vi "Dashboard Main.vi"() -> ()   [LabVIEW 2018]
uses:
  <vilib>/Utility/miscctls.llb/LVRowAndColumnTypeDef.ctl
  <vilib>/event_ctls.llb/eventvkey.ctl
  <vilib>/Rock Robotics/Network Tables/NT Read Boolean Array.vi
  <vilib>/Rock Robotics/Network Tables/NT Read Numeric Array.vi
  <vilib>/Rock Robotics/Network Tables/NT Write Numeric Array.vi
  <vilib>/Rock Robotics/Network Tables/NT Write Boolean.vi
  <vilib>/Rock Robotics/Network Tables/NT Write String Array.vi
  <vilib>/Rock Robotics/WPI/Dashboard/WPI_DashboardLogging Global.vi
panel:
  in  "Camera Name":string(combo)="No Camera Selection"
  in  "Camera Settings Right":T1={"Frame Rate"=30, "Compression"=30, "Size"=1, "DB Camera Config"=FALSE} {"Frame Rate" scale=1.0..30.0; "Compression" scale=100.0..-1.0; "Size" items=["640x480", "320x240", "160x120"]}
  in  "Camera Name Right":string(combo)="No Camera Selection"
  out "Camera Perf":string
  in  "Camera Settings":T1={"Frame Rate"=30, "Compression"=30, "Size"=1, "DB Camera Config"=FALSE} {"Frame Rate" scale=1.0..30.0; "Compression" scale=100.0..-1.0; "Size" items=["640x480", "320x240", "160x120"]}
  in  "TCP":refnum<k5>
  in  "Rec Mode":enum32{"Stop", "Record", "Playback"}(radio)
  out "Robot IP":string
  out "Image Message":string="Timeout in Camera Communications"
  in  "Dashboard Tab":T2(tab)
  out "SideOfFieldIndicator":bool
  in  "Side of Field:":string(combo)
  in  "Camera Lights Off:":bool
  out "Error Message:":string
  in  "Run Automated:":bool
  out "NT Connection":bool
  out "Mode":T3(ring)=enum."Auto Disabled"
  out "Right Camera Perf":cluster{"Bandwidth (Mbps)":dbl, "FPS":dbl}
  out "Front Left Setpoint:":dbl(knob)
  out "Front Right Setpoint:":dbl(knob)
  out "Back Left Setpoint:":dbl(knob)
  out "Back Right Setpoint:":dbl(knob)
  out "Reversed Modules":bool[](array[boolean])
  in  "Write Swerve Offsets:":bool
  in  "Task:":string(combo)
  out "PositionIndicator":bool
  out "TaskIndicator":bool
  in  "Start Position:":string(combo)
  out "Camera Image Right":T4(plugin-control)
  in  "CheckList":i32(listbox)
  in  "Test Slider":dbl(slide) scale=0.0..100.0 scale format="%#_3g"
  in  "On/Off":bool caption="Solenoid"
  in  "Test Name":u16(ring) items=["Select the test to run..."]
  in  "Test Tree":string(tree)
  in  "Motor":cluster{"Value":dbl, "Enable":bool} {"Value" scale=-1.0..1.0 scale format="%#_3g"}
  out "Progress":T5 {"Test Progress" scale=0.0..100.0}
  in  "Rev/Fwd":cluster{"Forward":bool, "Reverse":bool}
  in  "Test Ring":u16(ring) items=["Monochrome", "Color"]
  out "Cmd Status":string
  in  "Execute Command":bool
  in  "Command Params":string[][](table)
  in  "Command Selection":i32(listbox)
  out "Tree":string(tree)
  out "Camera Image":T4(plugin-control)
  out "Background":bool
  # "HW"
  # "HW"
  # "Swerve Modules:"
  # "Sandstorm Options:"
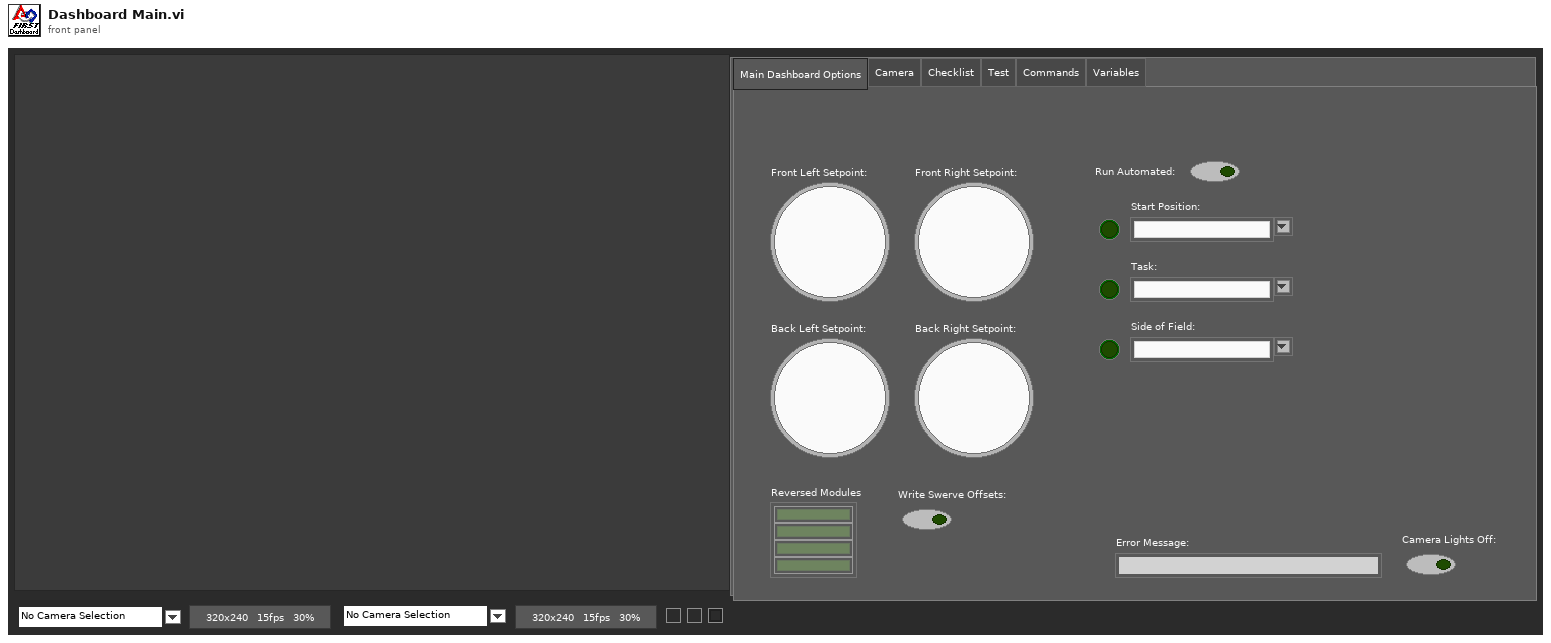
[diagram p1: front panel]
types:
  T1 = cluster{"Frame Rate":i32, "Compression":i32, "Size":u16, "DB Camera Config":bool}
  T2 = enum32{"Main Dashboard Options", "Camera", "Checklist", "Test", "Commands", "Variables"}
  T3 = enum8{"Tele-Op Disabled", "Tele-Op Enabled", "Auto Disabled", "Auto Enabled", "Test Disabled", "Test Enabled", "Disconnected", "No Code", "E-Stop"}
  T4 = typedef "IMAQ Image.ctl" = refnum<image>
  T5 = cluster{"Test Progress":u8, "Test Progress Text":string}
  T6 = cluster{"Save Path":path, "Interval (s)":dbl, "Keep":i32}
  T7 = enum32{"Drive", "Camera", "Basic", "Custom", "Test", "Commands", "Checklist", "Variables"}
  T8 = typedef "Image Type" = u32
  T9 = cluster{"IDs":cluster{"RPC field ID":u16, "Unique ID":u16}, "String":string}
  T10 = enum16{"open", "replace", "create", "open or create", "replace or create", "replace or create with confirmation"}
  T11 = cluster{"Error Strings":string, "Disable Counts":cluster{u16, u16}, "Rail Faults":cluster{u16, u16, u16}, "Robot IP":string, "DB Mode":u8, "Event Info":cluster{"Name":string, "Type":u8, "Number":u16, "Replay":u8}}
  T12 = cluster{"Storage":cluster{"Disk Free":u64, "RAM Block":u32, "RAM free":u32}, "CPU Utilization":cluster{"CPU % ISR":sgl, "CPU % Time Crit":sgl, "CPU % Timed Str":sgl, "CPU % High":sgl, "CPU % Above":sgl, "CPU % Normal":sgl, "CPU % Low":sgl}, "CAN":cluster{"% Bus Utilization":sgl, "Bus Off Cnt":u32, "TX_FIFO Full Cnt":u32, "Receive Error Cnt":u8, "Transmit Error Cnt":u8}, "HID":cluster{"HID Outputs":u32, "Rumble Low":u16, "Rumble High":u16}[]}
  T13 = cluster{"Status bits":cluster{"Test Mode":bool, "Autonomous":bool, "Enabled":bool, "Code Start":bool, "Brownout":bool, "Reserved 2":bool, "Reserved 3":bool, "E-Stop":bool}, "Code Trace":cluster{"Disabled":bool, "TeleOp":bool, "Auto":bool, "Test":bool}, "Controller Type":enum16{"unknown", "cRIO", "roboRio"}, "Code?":enum16{"unknown", "noCode", "code"}, "Battery V":dbl}
  T14 = cluster{"Control Bits":cluster{"TestMode":bool, "Autonomous":bool, "Enabled":bool, "FMS Present":bool, bool, bool, bool, "E-Stop":bool}, "Team Station ":u8, "Countdown":sgl, "Joystick Values":cluster{"Axes":dbl[], "Buttons":bool[], "POVs":i16[]}[]}
  T15 = cluster{"Camera Image":refnum<vi>, "Dashboard Tab":refnum<vi>, "Background":refnum<vi>, "Rec Mode":refnum<vi>, "Test Slider":refnum<vi>, "On/Off ":refnum<vi>, "Test Ring":refnum<vi>, "Rev/Fwd":refnum<vi>, "Test Name":refnum<vi>, "Motor":refnum<vi>, "Progress":refnum<vi>, "CheckList":refnum<vi>, "Tree":refnum<vi>, "Test Tree":refnum<vi>, "Command Params":refnum<vi>, "Command Selection":refnum<vi>, "Execute Command":refnum<vi>, "Cmd Status":refnum<vi>, "Camera Settings":refnum<vi>, "Camera Name":refnum<vi>, "Camera Perf":refnum<vi>, "Camera Settings Right":refnum<vi>, "Camera Name Right":refnum<vi>, "Camera Image Right":refnum<vi>}
  T16 = cluster{"Global Rectangle":i32[], "Contours":cluster{"Contour Type":u32, "ROI Type":u32, "Points":i32[]}[]}
  T17 = cluster{"Camera Name":string, string, "Saved DB Images Info":cluster{"Save Path":path, "Interval (s)":dbl, "Keep":i32}}
  T18 = cluster{"Camera Name Right":string, string, "Saved DB Images Info":cluster{"Save Path":path, "Interval (s)":dbl, "Keep":i32}}
  T19 = cluster{"Operation":enum16{"Update", "Clear"}, "Color Box":u32}[]
  T20 = typedef "eventvkey.ctl" = enum16{"ASCII", "Enter", "Return", "Shift", "Ctrl", "Alt", "Cmd", "Opt", "Caps", "NumLock", "Clear", "Break", "Up", "Down", "Left", "Right", "Insert", "Delete", "Home", "End", "PageUp", "PageDown", "Escape", "Help", "Pause", "ScrollLock", "F1", "F2", "F3", "F4", "F5", "F6", "F7", "F8", "F9", "F10", "F11", "F12", "F13", "F14", "F15", "F16", "F17", "F18", "F19", "F20", "F21", "F22", "F23", "F24", "Play", "VolumeUp", "VolumeDown", "Mute", "Two Byte Char"}
  T21 = cluster{"Image Size":bool, "Image Type":bool, "Pixel Value":bool, "ROI Information":bool, "Zoom Factor":bool}
  T22 = cluster{"Operation":enum16{"Update", "Clear"}, "Color Box":u32}
  T23 = typedef "LVRowAndColumnTypeDef.ctl" = cluster{"Row":i32, "Column":i32}
  T24 = cluster{"Shift":bool, "Ctrl":bool, "Alt":bool, "Cmd":bool, "Opt":bool}
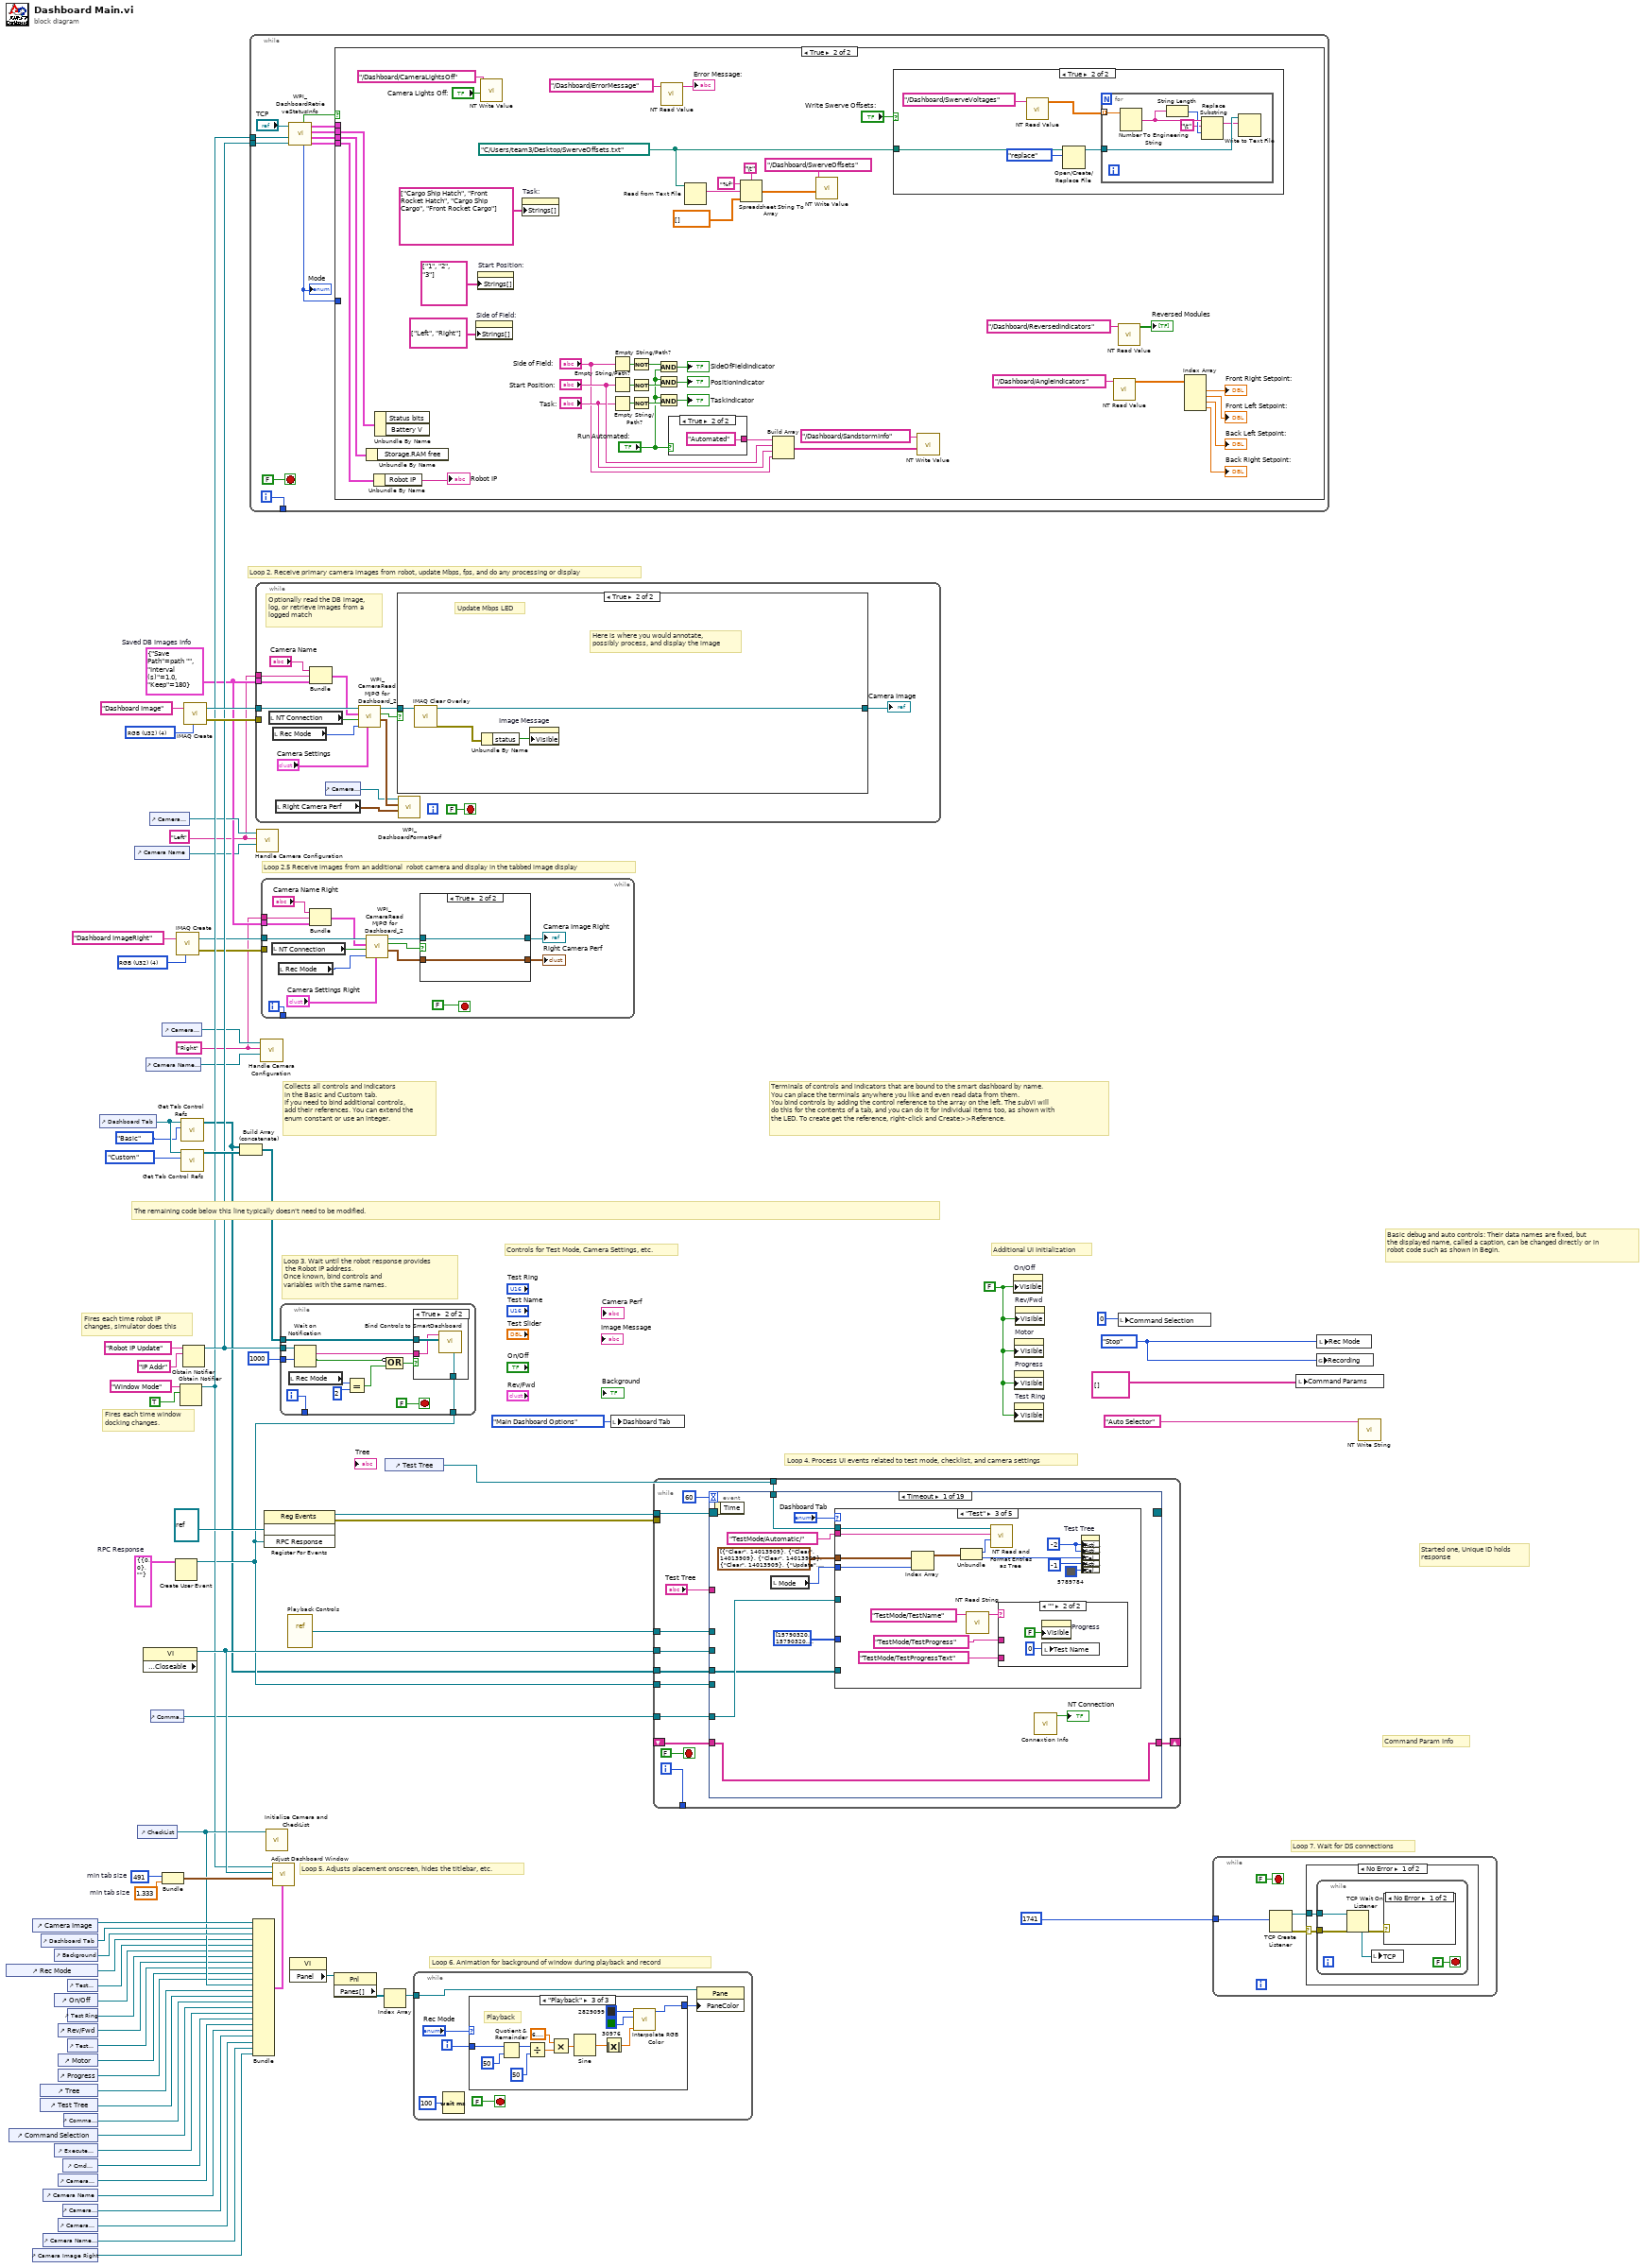
[diagram p0: block diagram]
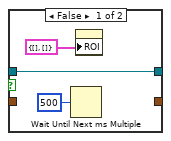
[diagram p2: hidden frame]
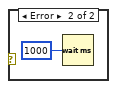
[diagram p3: hidden frame]
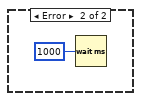
[diagram p4: hidden frame]
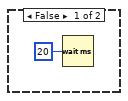
[diagram p5: hidden frame]
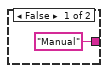
[diagram p6: hidden frame]
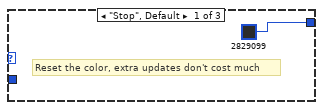
[diagram p8: hidden frame]
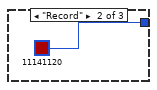
[diagram p9: hidden frame]
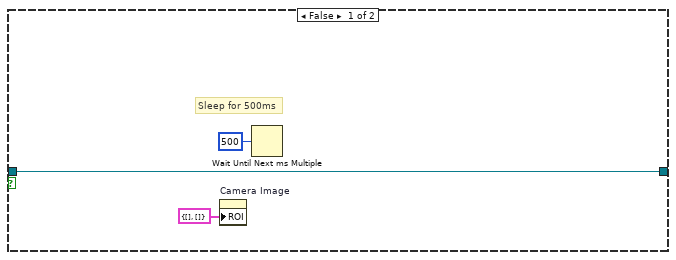
[diagram p11: hidden frame]
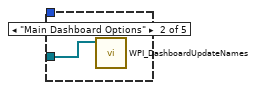
[diagram p13: hidden frame]
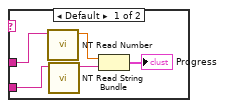
[diagram p14: hidden frame]
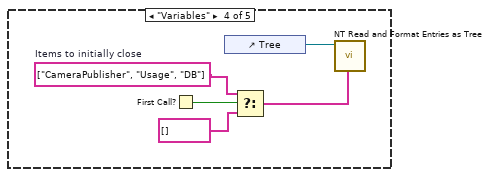
[diagram p15: hidden frame]
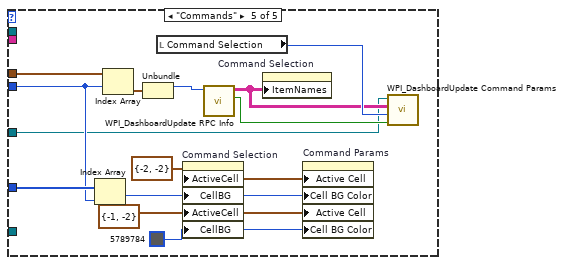
[diagram p16: hidden frame]
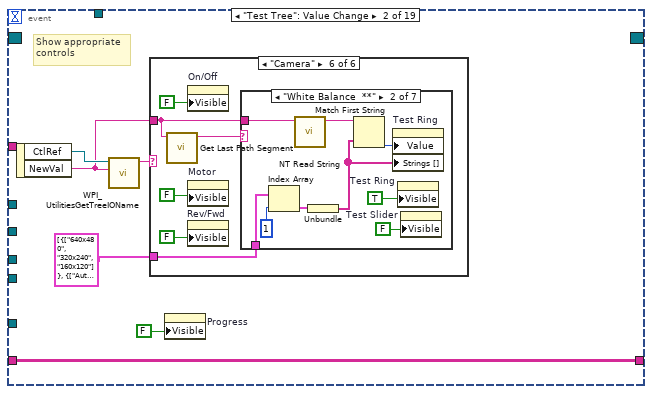
[diagram p17: hidden frame]
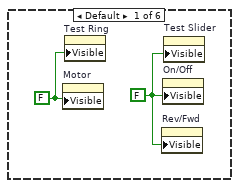
[diagram p18: hidden frame]
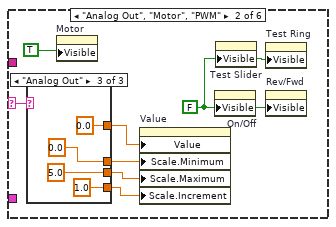
[diagram p19: hidden frame]
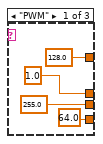
[diagram p20: hidden frame]
diagram:
  w6 = T6 {"Save Path"=path "", "Interval (s)"=1.0, "Keep"=180}  # Saved DB Images Info
  w5 = "Right"
  w4 = "Left"
  w16 = T8 4 items=["Grayscale (U8)", "Grayscale (I16)", "Grayscale (SGL)", "Complex (CSG)", "RGB (U32)", "HSL (U32)", "RGB (U64)"] ("Image Type")
  w29 = T9 {"IDs"={"RPC field ID"=0, "Unique ID"=0}, "String"=""}  # RPC Response
  w51 = 491  # min tab size
  w50 = 1.333  # min tab size
  w58 = enum32{"Stop", "Record", "Playback"}."Stop" ("Rec Mode")
  w35 = FALSE ("Visible")
  w75 = T8 4 items=["Grayscale (U8)", "Grayscale (I16)", "Grayscale (SGL)", "Complex (CSG)", "RGB (U32)", "HSL (U32)", "RGB (U64)"] ("Image Type")
  # "Loop 2.5 Receive images from an additional  robot camera and display in the tabbed image display"
  # "Command Param Info"
  # "Started one, Unique ID holds\nresponse"
  # "Loop 7. Wait for DS connections"
  # "Basic debug and auto controls: Their data names are fixed, but\nthe displayed name, called a caption, can be changed directly or in\nrobot code such as shown in Begin."
  # "Controls for Test Mode, Camera Settings, etc."
  # "Additional UI Initialization"
  # "Loop 6. Animation for background of window during playback and record"
  # "Fires each time robot IP\nchanges, simulator does this"
  # "Fires each time window\ndocking changes."
  # "Collects all controls and indicators\nin the Basic and Custom tab.\nIf you need to bind additional controls,\nadd their references. You can extend the\nenum constant or use an integer."
  # "The remaining code below this line typically doesn't need to be modified."
  # "Loop 4. Process UI events related to test mode, checklist, and camera settings"
  # "Terminals of controls and indicators that are bound to the smart dashboard by name.\nYou can place the terminals anywhere you like and even read data from them.\nYou bind controls by adding the control reference to the array on the left. The subVI will\ndo this for the contents of a tab, and you can do it for individual items too, as shown with\nthe LED. To create get the reference, right-click and Create>>Reference."
  # "Loop 3. Wait until the robot response provides\n the Robot IP address.\nOnce known, bind controls and\nvariables with the same names."
  # "Loop 5. Adjusts placement onscreen, hides the titlebar, etc."
  # "Loop 2. Receive primary camera images from robot, update Mbps, fps, and do any processing or display"
  n1 = control-ref of="Rec Mode"() -> (w41:refnum<vi>)
  n2 = control-ref of="Command Selection"() -> (w28:refnum<vi>)
  n3 = control-ref of="Camera Image"() -> (w53:refnum<vi>)
  n4 = control-ref of="Camera Image Right"() -> (w9:refnum<vi>)
  n5 = control-ref of="Tree"() -> (w45:refnum<vi>)
  n6 = control-ref of="Test Tree"() -> (w44:refnum<vi>)
  n7 = control-ref of="Dashboard Tab"() -> (w52:refnum<vi>)
  n8 = control-ref of="Camera Name"() -> (w2:refnum<vi>)
  n9 = control-ref of="Camera Name Right"() -> (w10:refnum<vi>)
  n10 = control-ref of="Background"() -> (w48:refnum<vi>)
  n11 = control-ref of="On/Off"() -> (w39:refnum<vi>)
  n12 = control-ref of="Execute Command"() -> (w30:refnum<vi>)
  n13 = control-ref of="Rev/Fwd"() -> (w37:refnum<vi>)
  n14 = control-ref of="Motor"() -> (w42:refnum<vi>)
  n15 = control-ref of="Progress"() -> (w36:refnum<vi>)
  n16 = control-ref of="Camera Settings"() -> (w21:refnum<vi>)
  n17 = control-ref of="Camera Settings Right"() -> (w11:refnum<vi>)
  n18 = control-ref of="Cmd Status"() -> (w24:refnum<vi>)
  n19 = control-ref of="Camera Perf"() -> (w20:refnum<vi>)
  n20 = control-ref of="Command Params"() -> (w31:refnum<vi>)
  n21 = control-ref of="Test Slider"() -> (w40:refnum<vi>)
  n22 = control-ref of="Test Ring"() -> (w38:refnum<vi>)
  n23 = control-ref of="Test Name"() -> (w43:refnum<vi>)
  n24 = control-ref of="Dashboard Tab"() -> (w56:refnum<vi>)
  n25 = control-ref of="Camera Name"() -> (w3:refnum<vi>)
  n26 = control-ref of="CheckList"() -> (w46:refnum<vi>)
  n27 = property class="VI" props=["Front Panel.Closeable"]() -> (reference out=w57:refnum<vi>)  [unwired: 2 in, 2 out]
  n28 = control-ref of="Camera Name Right"() -> (w12:refnum<vi>)
  n29 = control-ref of="Camera Settings"() -> (w22:refnum<vi>)
  n30 = control-ref of="Command Params"() -> (w23:refnum<vi>)
  n31 = control-ref of="Camera Settings Right"() -> (w13:refnum<vi>)
  n32 = Bundle("min tab size"=w51, "min tab size"=w50) -> (w49:cluster{"min tab size":i32, "min tab size":dbl})  [unwired: 1 in]
  n33 = Create User Event(user event datatype=w29) -> (user event=w25:refnum<user-event>)  [unwired: 1 in, 1 out]
  n34 = call "IMAQ Create"("Image Name"="Dashboard ImageRight", "Image Type"=w16) -> ("New Image"=w15:T4, "error out"=w14:errorcluster)  [unwired: 2 in, 1 out]
  n35 = Obtain Notifier(name (unnamed)="Window Mode", notification data type=TRUE) -> (notifier out=w33:refnum<notifier>)  [unwired: 2 in, 2 out]
  n36 = call <vilib>:"Get Tab Control Refs.vi"("Page Index"=T7."Basic" ("Dashboard Tab"), "TabControl in"=w56) -> ("ControlsOnPage"=w19:refnum<vi>[])  [unwired: 9 in]
  n37 = call <vilib>:"Get Tab Control Refs.vi"("Page Index"=T7."Custom" ("Dashboard Tab"), "TabControl in"=w56) -> ("ControlsOnPage"=w55:refnum<vi>[])  [unwired: 9 in]
  n38 = Obtain Notifier(name (unnamed)="Robot IP Update", notification data type="IP Addr" ("name (unnamed)")) -> (notifier out=w34:refnum<notifier>)  [unwired: 2 in, 2 out]
  n39 = call "IMAQ Create"("Image Name"="Dashboard Image", "Image Type"=w75) -> ("New Image"=w73:T4, "error out"=w72:errorcluster)  [unwired: 2 in, 1 out]
  n40 = Build Array (concatenate)(w19, w55) -> (w54:refnum<vi>[])
  n41 = while {
    tunnel: [w85] -> _
    tunnel: w34 -> [w79]
    tunnel: w33 -> [w76]
    i -> [w85]
    stop <- FALSE stop-if-true
    n42 = call <vilib>:"WPI_DashboardRetrieveStatusInfo.vi"("Binding Refnum"=w79, "Window Mode Notifier"=w76, "TCP Cnx"="TCP") -> ("Power and Errors"=w80:T11, "Robot Metrics"=w83:T12, "Status Info"=w84:T13, "Control Info"=w81:T14, "Robot Mode"=w78:T3, "Process?"=w82:bool)  [unwired: 3 in]
    "Mode" <- w78
    n43 = case shown="True" w82 {
      tunnel: w84 -> [_ w130]
      tunnel: w83 -> [_ w129]
      tunnel: w81 -> [_ _]
      tunnel: w80 -> [_ w128]
      tunnel: w78 -> [_ _]
      frame False {
        n44 = Wait (ms)(milliseconds to wait=u32 20) -> ()  [unwired: 1 out]
      }
      frame True {
        w110 = path "C:/Users/team3/Desktop/SwerveOffsets.txt" ("file (use dialog)")
        n45 = Unbundle By Name(w129) -> ()  [unwired: 1 out]
        n46 = Unbundle By Name(w128) -> ("Robot IP"=→"Robot IP":string)
        n47 = Unbundle By Name(w130) -> ()  [unwired: 2 out]
        n48 = property on="Side of Field:" class="CmbBox"("Strings[]"=string[] ["Left", "Right"]) -> ()  [unwired: 2 in, 2 out]
        n49 = property on="Start Position:" class="CmbBox"("Strings[]"=string[] ["1", "2", "3"]) -> ()  [unwired: 2 in, 2 out]
        n50 = call-poly <vilib>:"NT Write Value.vi"("Boolean"="Camera Lights Off:", "Name"="/Dashboard/CameraLightsOff") -> ()  [unwired: 9 in, 1 out]
        n51 = property on="Task:" class="CmbBox"("Strings[]"=string[] ["Cargo Ship Hatch", "Front Rocket Hatch", "Cargo Ship Cargo", "Front Rocket Cargo"]) -> ()  [unwired: 2 in, 2 out]
        n52 = Empty String/Path?(string/path="Side of Field:") -> (empty?=w91:bool)
        n53 = Empty String/Path?(string/path="Start Position:") -> (empty?=w106:bool)
        n54 = Empty String/Path?(string/path="Task:") -> (empty?=w103:bool)
        n55 = Not(x=w91) -> (.not. x?=w89:bool)
        n56 = Not(x=w106) -> (.not. x?=w105:bool)
        n57 = Not(x=w103) -> (.not. x?=w104:bool)
        n58 = And(x=w89, y="Run Automated:") -> (x .and. y?=→"SideOfFieldIndicator":bool)
        n59 = And(x="Run Automated:", y=w105) -> (x .and. y?=→"PositionIndicator":bool)
        n60 = And(x="Run Automated:", y=w104) -> (x .and. y?=→"TaskIndicator":bool)
        n61 = call-poly <vilib>:"NT Read Value.vi"("Name"="/Dashboard/ErrorMessage") -> ("String"=→"Error Message:":string)  [unwired: 9 in, 1 out]
        n62 = case shown="True" "Run Automated:" {
          tunnel: ["Manual" "Automated"] -> w100
          frame False {
          }
          frame True {
          }
        }
        n63 = Read from Text File(file (use dialog)=w110) -> (text=w124:string)  [unwired: 3 in, 3 out]
        n64 = Spreadsheet String To Array(delimiter (Tab)="\t", format string="%f", spreadsheet string=w124, array type (2D Dbl)=dbl[] []) -> (array=w123:dbl[])
        n65 = Build Array(w100, "Start Position:", "Task:", "Side of Field:") -> (w107:string[])
        n66 = call-poly <vilib>:"NT Write Value.vi"("Numeric Array"=w123, "Name"="/Dashboard/SwerveOffsets") -> ()  [unwired: 9 in, 1 out]
        n67 = case shown="True" "Write Swerve Offsets:" {
          tunnel: w110 -> [_ w134]
          frame False {
          }
          frame True {
            n68 = call-poly <vilib>:"NT Read Value.vi"("Name"="/Dashboard/SwerveVoltages") -> ("Numeric Array"=w133:dbl[])  [unwired: 9 in, 1 out]
            n69 = Open/Create/Replace File(file path (use dialog)=w134, operation (0:open)=T10."replace") -> (refnum out=w136:refnum<file>)  [unwired: 4 in, 2 out]
            n70 = for {
              tunnel: w136 -> [w142]
              tunnel: w133 -> [w143] mode=indexing
              n71 = Number To Engineering String(4:w143) -> (0:w141:string)  [unwired: 3 in]
              n72 = String Length(string=w141) -> (length=w140:i32)
              n73 = Replace Substring(3:w140, 4:"\t", 5:w141) -> (1:w138:string)  [unwired: 1 in, 1 out]
              n74 = Write to Text File(file (use dialog)=w142, text=w138) -> ()  [unwired: 2 in, 3 out]
            }
          }
        }
        n75 = call-poly <vilib>:"NT Write Value.vi"("String Array"=w107, "Name"="/Dashboard/SandstormInfo") -> ()  [unwired: 9 in, 1 out]
        n76 = call-poly <vilib>:"NT Read Value.vi"("Name"="/Dashboard/AngleIndicators") -> ("Numeric Array"=w115:dbl[])  [unwired: 9 in, 1 out]
        n77 = call-poly <vilib>:"NT Read Value.vi"("Name"="/Dashboard/ReversedIndicators") -> ("Boolean Array"=→"Reversed Modules":bool[])  [unwired: 9 in, 1 out]
        n78 = Index Array(array=w115) -> (element #1=→"Front Right Setpoint:":dbl, element #2=→"Front Left Setpoint:":dbl, element #3=→"Back Left Setpoint:":dbl, element #4=→"Back Right Setpoint:":dbl)  [unwired: 4 in]
      }
    }
  }
  n79 = Bundle("Camera Image"=w53, "Dashboard Tab"=w52, "Background"=w48, "Rec Mode"=w41, "Test Slider"=w40, "On/Off"=w39, "Test Ring"=w38, "Rev/Fwd"=w37, "Test Name"=w43, "Motor"=w42, "Progress"=w36, "CheckList"=w46, "Tree"=w45, "Test Tree"=w44, "Command Params"=w31, "Command Selection"=w28, "Execute Command"=w30, "Cmd Status"=w24, "Camera Settings"=w21, "Camera Name"=w2, "Camera Perf"=w20, "Camera Settings Right"=w11, "Camera Name Right"=w10, "Camera Image Right"=w9) -> (w47:T15)  [unwired: 1 in]
  n80 = while {
    tunnel: w73 -> [w157]
    tunnel: w72 -> [_]
    tunnel: w6 -> [w150]
    tunnel: w4 -> [w148]
    stop <- FALSE stop-if-true
    # "Optionally read the DB image,\nlog, or retrieve images from a\nlogged match"
    n81 = local read "NT Connection"() -> (w151:bool)
    n82 = local read "Rec Mode"() -> (w154:enum32{"Stop", "Record", "Playback"})
    n83 = local read "Right Camera Perf"() -> (w146:cluster{"Bandwidth (Mbps)":dbl, "FPS":dbl})
    n84 = Bundle("Camera Name"="Camera Name", w148, "Saved DB Images Info"=w150) -> (w149:T17)  [unwired: 1 in]
    n85 = control-ref of="Camera Perf"() -> (w145:refnum<vi>)
    n86 = call <vilib>:"WPI_CameraRead MJPG for Dashboard_2.vi"("Camera Settings"="Camera Settings", "Rec Mode"=w154, "NT Connection"=w151, "Capture Info"=w149, "Image in"=w157) -> ("perf info"=w147:cluster{"Bandwidth (Mbps)":dbl, "fps":dbl}, "Active"=w155:bool, "Image\\ out"=w156:T4)  [unwired: 4 in]
    n87 = case shown="True" w155 {
      tunnel: w156 -> [w160 w163]
      tunnel: [w160 w162] -> w152
      frame False {
        # "Sleep for 500ms"
        n88 = property on="Camera Image" class="ImageControl"("ROI"=T16 {"Global Rectangle"=[], "Contours"=[]}) -> ()  [unwired: 2 in, 2 out]
        n89 = Wait Until Next ms Multiple(millisecond multiple=u32 500) -> ()  [unwired: 1 out]
      }
      frame True {
        # "Here is where you would annotate,\npossibly process, and display the image"
        # "Update Mbps LED"
        n90 = call "IMAQ Clear Overlay"("Image"=w163) -> ("error out"=w164:errorcluster, "Image Out"=w162:T4)  [unwired: 2 in, 7 out]
        n91 = Unbundle By Name(w164) -> ("status"=w165:bool)
        n92 = property on="Image Message" class="Str"("Visible"=w165) -> ()  [unwired: 2 in, 2 out]
      }
    }
    "Camera Image" <- w152
    n93 = call <vilib>:"WPI_DashboardFormatPerf.vi"("Right Camera Perf"=w146, "Performance"=w147, "String in"=w145) -> ()  [unwired: 9 in]
  }
  n94 = call "Handle Camera Configuration.vi"("CameraNameRef"=w3, "Display Name"=w4, "ClusterRef"=w22) -> ()  [unwired: 9 in]
  n95 = call "Handle Camera Configuration.vi"("CameraNameRef"=w12, "Display Name"=w5, "ClusterRef"=w13) -> ()  [unwired: 9 in]
  n96 = while {
    tunnel: w15 -> [w180]
    tunnel: w14 -> [_]
    tunnel: [w175] -> _
    tunnel: w6 -> [w171]
    tunnel: w5 -> [w168]
    i -> [w175]
    stop <- FALSE stop-if-true
    n97 = local read "NT Connection"() -> (w172:bool)
    n98 = local read "Rec Mode"() -> (w179:enum32{"Stop", "Record", "Playback"})
    n99 = Bundle("Camera Name Right"="Camera Name Right", w168, "Saved DB Images Info"=w171) -> (w170:T18)  [unwired: 1 in]
    n100 = call <vilib>:"WPI_CameraRead MJPG for Dashboard_2.vi"("Camera Settings"="Camera Settings Right", "Rec Mode"=w179, "NT Connection"=w172, "Capture Info"=w170, "Image in"=w180) -> ("perf info"=w166:cluster{"Bandwidth (Mbps)":dbl, "fps":dbl}, "Active"=w174:bool, "Image\\ out"=w177:T4)  [unwired: 4 in]
    n101 = case shown="True" w174 {
      tunnel: w177 -> [w182 w185]
      tunnel: [w182 w185] -> w173
      tunnel: [_ w184] -> w167
      tunnel: w166 -> [_ w184]
      frame False {
        n102 = Wait Until Next ms Multiple(millisecond multiple=u32 500) -> ()  [unwired: 1 out]
        n103 = property on="Camera Image Right" class="ImageControl"("ROI"=T16 {"Global Rectangle"=[], "Contours"=[]}) -> ()  [unwired: 2 in, 2 out]
      }
      frame True {
      }
    }
    "Camera Image Right" <- w173
    "Right Camera Perf" <- w167
  }
  n104 = register-events(refnum<vi> refnum, w25) -> (reference out=w62:refnum<event-registration>, error out=w61:errorcluster)  [unwired: 2 in]
  n105 = call "Initialize Camera and CheckList.vi"("ListBox in"=w46) -> ()  [unwired: 11 in]
  n106 = call "Adjust Dashboard Window.vi"("Sizing Refnums"=w47, "Size Constraints"=w49, "VI"=w57, "WIn Mode"=w33) -> ()  [unwired: 8 in]
  n107 = while {
    tunnel: w54 -> [w197]
    tunnel: w34 -> [w195]
    tunnel: [w193] -> _
    tunnel: u32 1000 ("milliseconds to wait") -> [w192]
    tunnel: w25 -> [w186]
    i -> [w193]
    stop <- FALSE stop-if-true
    n108 = local read "Rec Mode"() -> (w188:enum32{"Stop", "Record", "Playback"})
    n109 = Wait on Notification(notifier=w195, timeout in ms (-1)=w192) -> (notification=w194:string, timed out?=w190:bool)  [unwired: 2 in, 2 out]
    n110 = Equal?(x=w188, y=u16 2 ("Rec Mode")) -> (x = y?=w189:bool)
    n111 = Compound Arithmetic op=OR(invert w190, w189) -> (w191:bool)
    n112 = case shown="True" w191 {
      tunnel: w197 -> [_ w200]
      tunnel: w194 -> [_ w199]
      tunnel: w186 -> [_ w198]
      frame False {
      }
      frame True {
        n113 = call <vilib>:"Bind Controls to SmartDashboard.vi"("RPC ref"=w198, "Bound Control Refs"=w200, "Server IP Address"=w199) -> ()  [unwired: 9 in]
      }
    }
  }
  n114 = vi-ref "Playback Controls.vi"() -> (w63:refnum<vi>)
  n115 = property class="VI"() -> ("Panel"=w65:refnum<vi>)  [unwired: 2 in, 2 out]
  n116 = property class="Pnl"(reference=w65) -> ("Panes[]"=w66:refnum<vi>[])  [unwired: 1 in, 2 out]
  n117 = Index Array(array=w66) -> (element=w64:refnum<vi>)  [unwired: 1 in]
  n118 = control-ref of="Test Tree"() -> (w67:refnum<vi>)
  n119 = while {
    tunnel: w64 -> [w202]
    i -> [w205]
    stop <- FALSE stop-if-true
    n120 = Wait (ms)(milliseconds to wait=u32 100) -> ()  [unwired: 1 out]
    n121 = case shown="\"Playback\"" "Rec Mode" {
      tunnel: w205 -> [_ _ w220]
      tunnel: [u32 2829099 ("Base Color") u32 11141120 ("Target Color") w209] -> w201
      frame "Stop", Default {
        # "Reset the color, extra updates don't cost much"
      }
      frame "Record" {
      }
      frame "Playback" {
        # "Playback"
        n122 = Quotient & Remainder(x=w220, y=u32 50 ("milliseconds to wait")) -> (x-y*floor(x/y)=w216:u32)  [unwired: 1 out]
        n123 = Divide(x=w216, y=u32 50 ("milliseconds to wait")) -> (x/y=w213:dbl)
        n124 = Multiply(x=6.283185307179586, y=w213) -> (x*y=w218:dbl)
        n125 = Sine(x=w218) -> (sin(x)=w217:dbl)
        n126 = Absolute Value(x=w217) -> (abs(x)=w210:dbl)
        n127 = call "Interpolate RGB Color.vi"("Proportion"=w210, "Target Color"=u32 30976, "Base Color"=u32 2829099) -> ("Result Color"=w209:u32)  [unwired: 8 in]
      }
    }
    n128 = property class="Pane"(reference=w202, "PaneColor"=w201) -> ()  [unwired: 1 in, 2 out]
  }
  n129 = local write "Dashboard Tab"(T2."Main Dashboard Options" ("Dashboard Tab")) -> ()
  n130 = while {
    tunnel: [w230] -> _
    tunnel: w67 -> [w229]
    tunnel: w63 -> [w228]
    tunnel: w62 -> [w227]
    tunnel: w61 -> [_]
    tunnel: w57 -> [w226]
    tunnel: w25 -> [w225]
    tunnel: w23 -> [w224]
    shift-right: [w223] -> _
    shift-left: _ -> [w222]
    tunnel: w19 -> [w221]
    i -> [w230]
    stop <- FALSE stop-if-true
    n131 = event shown="[0] Timeout" {
      selector: w227 -> [_ _ _ _ _ _ _ _ _ _ _ _ _ _ _ _ _ _ _]
      dyn-events: [_ _ _ _ _ _ _ _ _ _ _ _ _ _ w484 _ _ _ _] -> _
      timeout: u32 60 ("milliseconds to wait") -> [_ _ _ _ _ _ _ _ _ _ _ _ _ _ _ _ _ _ _]
      tunnel: w229 -> [w242 _ _ _ _ _ _ _ _ _ _ _ _ _ _ _ _ _ _]
      tunnel: "Test Tree" -> [_ _ _ _ _ _ _ _ _ w451 w459 w461 w465 w473 _ _ _ _ _]
      tunnel: w228 -> [_ _ _ _ _ _ _ _ _ _ _ _ _ _ w486 _ w504 _ _]
      tunnel: w226 -> [_ _ _ _ _ _ _ _ _ _ _ _ _ _ w482 _ _ _ _]
      tunnel: w225 -> [_ _ _ _ _ _ _ _ _ _ _ _ _ _ w480 _ _ _ _]
      tunnel: w224 -> [w237 _ _ _ w402 _ _ _ _ _ _ _ _ _ _ _ _ _ _]
      tunnel: [w236 w285 w387 w392 w400 w409 w419 w426 w438 w450 w457 w460 w464 w472 w479 w499 w501 w505 w518] -> w223
      tunnel: w222 -> [w236 w285 w387 w392 w400 _ _ w426 w438 w450 w457 w460 w464 w472 w479 w499 w501 w505 w518]
      tunnel: w221 -> [w234 _ _ _ _ _ _ _ _ _ _ _ _ _ _ _ _ _ _]
      event Timeout {
        n132 = event-data() -> ()  [unwired: 1 in, 1 out]
        n133 = local read "Mode"() -> (w239:T3)
        n134 = case shown="\"Test\"" "Dashboard Tab" {
          tunnel: w242 -> [_ _ w258 _ _]
          tunnel: "TestMode/Automatic/" ("Name Pattern") -> [_ _ w257 _ _]
          tunnel: T19 [{"Operation"=enum."Clear", "Color Box"=14013909}, {"Operation"=enum."Clear", "Color Box"=14013909}, {"Operation"=enum."Clear", "Color Box"=14013909}, {"Operation"=enum."Clear", "Color Box"=14013909}, {"Operation"=enum."Update", "Color Box"=14013909}, {"Operation"=enum."Update", "Color Box"=16777215}, {"Operation"=enum."Clear", "Color Box"=14013909}, {"Operation"=enum."Clear", "Color Box"=14013909}, {"Operation"=enum."Clear", "Color Box"=14013909}] -> [_ _ w250 _ w278]
          tunnel: w239 -> [_ _ w249 _ w277]
          tunnel: u32[] [15790320, 15790320, 15790320, 15790320, 16777215, 16777215, 15790320, 15790320, 15790320] -> [_ _ _ _ w283]
          tunnel: w237 -> [_ _ _ _ w271]
          tunnel: w234 -> [_ w244 _ _ _]
          frame "Camera", Default {
          }
          frame "Main Dashboard Options" {
            n135 = call <vilib>:"WPI_DashboardUpdateNames.vi"("Controls on Tab"=w244) -> ()  [unwired: 11 in]
          }
          frame "Test" {
            w256 = -2 ("Active Item:Row Number")
            n136 = Index Array(array=w250, index=w249) -> (element=w251:T22)
            n137 = Unbundle(w251) -> ("Operation"=w252:enum16{"Update", "Clear"}, "Color Box"=w253:u32)
            n138 = call <vilib>:"NT Read String.vi"("Name"="TestMode/TestName") -> ("String"=w247:string)  [unwired: 9 in, 1 out]
            n139 = call <vilib>:"NT Read and Format Entries as Tree.vi"("Operation"=w252, "Name Pattern"=w257, "Tree Refnum"=w258) -> ()  [unwired: 7 in, 2 out]
            n140 = case shown="\"\"" w247 {
              tunnel: "TestMode/TestProgress" ("Name") -> [w260 _]
              tunnel: "TestMode/TestProgressText" ("Name") -> [w259 _]
              frame Default {
                n141 = call <vilib>:"NT Read Number.vi"("Name"=w260) -> ("Numeric"=w261:dbl)  [unwired: 9 in, 1 out]
                n142 = call <vilib>:"NT Read String.vi"("Name"=w259) -> ("String"=w262:string)  [unwired: 9 in, 1 out]
                n143 = Bundle("Numeric"=w261, "String"=w262) -> (→"Progress":cluster{"Numeric":dbl, "String":string})  [unwired: 1 in]
              }
              frame "" {
                n144 = property on="Progress" class="Clust (strict)"("Visible"=FALSE) -> ()  [unwired: 2 in, 2 out]
                n145 = local write "Test Name"(u16 0) -> ()
              }
            }
            n146 = property on="Test Tree" class="Tree (strict)"("Active Item Row Number"=w256, "ActiveColNum"=w256, "CellBG"=w253, "Active Item Row Number"=-1 ("Active Item:Row Number"), "CellBG"=u32 5789784 ("Color Box")) -> ()  [unwired: 2 in, 2 out]
          }
          frame "Variables" {
            w268 = string[] ["CameraPublisher", "Usage", "DB"]  # Items to initially close
            n147 = First Call?() -> (First Call?: T/F=w269:bool)
            n148 = control-ref of="Tree"() -> (w270:refnum<vi>)
            n149 = Select(t=w268, s=w269, f=string[] []) -> (s? t:f=w266:string[])
            n150 = call <vilib>:"NT Read and Format Entries as Tree.vi"("Tags to  Close"=w266, "Tree Refnum"=w270) -> ()  [unwired: 8 in, 2 out]
          }
          frame "Commands" {
            w279 = u32 5789784 ("Color Box")
            w280 = T23 {"Row"=-1, "Column"=-2} ("Active Cell:Active Cell")
            w282 = T23 {"Row"=-2, "Column"=-2} ("Active Cell:Active Cell")
            n151 = Index Array(array=w283, index=w277) -> (element=w281:u32)
            n152 = Index Array(array=w278, index=w277) -> (element=w276:T22)
            n153 = Unbundle(w276) -> ("Operation"=w275:enum16{"Update", "Clear"})  [unwired: 1 out]
            n154 = local read "Command Selection"() -> (w274:i32)
            n155 = property on="Command Selection" class="MCListbox (strict)"("ActiveCell"=w282, "CellBG"=w281, "ActiveCell"=w280, "CellBG"=w279) -> ()  [unwired: 2 in, 2 out]
            n156 = call <vilib>:"WPI_DashboardUpdate RPC Info.vi"("Operation"=w275) -> ("update"=w273:bool, "commands"=w272:string[][])  [unwired: 9 in]
            n157 = property on="Command Selection" class="MCListbox (strict)"("ItemNames"=w272) -> ()  [unwired: 2 in, 2 out]
            n158 = property on="Command Params" class="Tbl (strict)"("Active Cell"=w282, "Cell BG Color"=w281, "Active Cell"=w280, "Cell BG Color"=w279) -> ()  [unwired: 2 in, 2 out]
            n159 = call <vilib>:"WPI_DashboardUpdate Command Params.vi"("Update"=w273, "NewVal"=w274, "Commands"=w272, "Param Tbl"=w271) -> ()  [unwired: 7 in, 1 out]
          }
        }
        n160 = call <vilib>:"Connextion Info.vi"() -> ("Connected"=→"NT Connection":bool)  [unwired: 10 in, 1 out]
      }
      event "Test Tree": Value Change {
        # "Show appropriate\ncontrols"
        n161 = event-data() -> ("CtlRef"=w288:refnum<vi>, "NewVal"=w286:string)  [unwired: 1 in]
        n162 = call <vilib>:"WPI_UtilitiesGetTreeIOName.vi"("NewVal"=w286, "TreeControl in"=w288) -> ("I/O Name"=w289:string)  [unwired: 9 in]
        n163 = case shown="\"Camera\"" w289 {
          selector: w289 -> [_ w296 _ w318 w327 _]
          tunnel: w286 -> [_ _ w315 w317 _ w334]
          tunnel: cluster{string[]}[] [{["640x480", "320x240", "160x120"]}, {["Auto", "Fixed indoor", "Fixed outdoor 1", "Fixed outdoor 2", "Fixed fluorescent 1", "Fixed fluorescent 2", "Hold current"]}, {["Auto", "Flicker-free 50 Hz", "Flicker-free 60 Hz", "Hold current"]}, {["None", "Prioritize frame rate", "Prioritize image quality"]}, {["Monochrome", "Color"]}] -> [_ _ _ _ _ w333]
          frame Default {
            w291 = FALSE ("Visible")
            w290 = FALSE ("Visible")
            n164 = property on="Motor" class="Clust (strict)"("Visible"=w290) -> ()  [unwired: 2 in, 2 out]
            n165 = property on="Test Ring" class="Ring (strict)"("Visible"=w290) -> ()  [unwired: 2 in, 2 out]
            n166 = property on="Rev/Fwd" class="Clust (strict)"("Visible"=w291) -> ()  [unwired: 2 in, 2 out]
            n167 = property on="On/Off" class="Bool (strict)"("Visible"=w291) -> ()  [unwired: 2 in, 2 out]
            n168 = property on="Test Slider" class="Slide (strict)"("Visible"=w291) -> ()  [unwired: 2 in, 2 out]
          }
          frame "Analog Out", "Motor", "PWM" {
            w297 = FALSE ("Visible")
            n169 = case shown="\"Analog Out\"" w296 {
              tunnel: [1.0 ("Value") -1.0 ("Value") 0.0 ("Value")] -> w295
              tunnel: [255.0 ("Value") 1.0 ("Value") 5.0 ("Value")] -> w294
              tunnel: [128.0 ("Value") 0.0 ("Value") 0.0 ("Value")] -> w293
              tunnel: [64.0 ("Value") 0.5 ("Value") 1.0 ("Value")] -> w292
              frame "PWM" {
              }
              frame "Motor", Default {
              }
              frame "Analog Out" {
              }
            }
            n170 = property on="Motor" class="Clust (strict)"("Visible"=TRUE) -> ()  [unwired: 2 in, 2 out]
            n171 = property on="Value" class="Slide (strict)"("Value"=w293, "Scale.Minimum"=w295, "Scale.Maximum"=w294, "Scale.Increment"=w292) -> ()  [unwired: 2 in, 2 out]
            n172 = property on="On/Off" class="Bool (strict)"("Visible"=w297) -> ()  [unwired: 2 in, 2 out]
            n173 = property on="Test Slider" class="Slide (strict)"("Visible"=w297) -> ()  [unwired: 2 in, 2 out]
            n174 = property on="Test Ring" class="Ring (strict)"("Visible"=w297) -> ()  [unwired: 2 in, 2 out]
            n175 = property on="Rev/Fwd" class="Clust (strict)"("Visible"=w297) -> ()  [unwired: 2 in, 2 out]
          }
          frame "Servo" {
            w313 = FALSE ("Visible")
            n176 = call <vilib>:"NT Read Number.vi"("Name"=w315) -> ("Numeric"=w314:dbl)  [unwired: 9 in, 1 out]
            n177 = property on="Test Slider" class="Slide (strict)"("Visible"=TRUE, "Scale.Maximum"=170.0 ("Scale.Range:Maximum")) -> ()  [unwired: 2 in, 2 out]
            n178 = local write "Test Slider"(w314) -> ()
            n179 = property on="Motor" class="Clust (strict)"("Visible"=w313) -> ()  [unwired: 2 in, 2 out]
            n180 = property on="Rev/Fwd" class="Clust (strict)"("Visible"=w313) -> ()  [unwired: 2 in, 2 out]
            n181 = property on="On/Off" class="Bool (strict)"("Visible"=w313) -> ()  [unwired: 2 in, 2 out]
            n182 = property on="Test Ring" class="Ring (strict)"("Visible"=w313) -> ()  [unwired: 2 in, 2 out]
          }
          frame "Relay", "Solenoid" {
            w316 = FALSE ("Visible")
            n183 = property on="Motor" class="Clust (strict)"("Visible"=w316) -> ()  [unwired: 2 in, 2 out]
            n184 = property on="Test Slider" class="Slide (strict)"("Visible"=w316) -> ()  [unwired: 2 in, 2 out]
            n185 = Search and Replace String(input string=w317, search string="/Value  **", replace string="/Direction") -> (result string=w323:string)  [unwired: 5 in, 3 out]
            n186 = property on="Test Ring" class="Ring (strict)"("Visible"=w316) -> ()  [unwired: 2 in, 2 out]
            n187 = call <vilib>:"NT Read String.vi"("Name"=w323) -> ("String"=w321:string)  [unwired: 9 in, 1 out]
            n188 = Equal?(x="Both directions", y=w321) -> (x = y?=w319:bool)
            n189 = Not(x=w319) -> (.not. x?=w320:bool)
            n190 = property on="Rev/Fwd" class="Clust (strict)"("Visible"=w319) -> ()  [unwired: 2 in, 2 out]
            n191 = property on="On/Off" class="Bool (strict)"("Visible"=w320, "Caption.Text"=w318) -> ()  [unwired: 2 in, 2 out]
          }
          frame "Compressor", "Digital Out" {
            w326 = FALSE ("Visible")
            # "Get direction and finish"
            n192 = property on="Motor" class="Clust (strict)"("Visible"=w326) -> ()  [unwired: 2 in, 2 out]
            n193 = property on="Test Slider" class="Slide (strict)"("Visible"=w326) -> ()  [unwired: 2 in, 2 out]
            n194 = property on="Test Ring" class="Ring (strict)"("Visible"=w326) -> ()  [unwired: 2 in, 2 out]
            n195 = property on="On/Off" class="Bool (strict)"("Visible"=TRUE, "Caption.Text"=w327) -> ()  [unwired: 2 in, 2 out]
            n196 = property on="Rev/Fwd" class="Clust (strict)"("Visible"=FALSE) -> ()  [unwired: 2 in, 2 out]
          }
          frame "Camera" {
            n197 = call <vilib>:"Get Last Path Segment.vi"("String in"=w334) -> ("String out"=w335:string)  [unwired: 10 in]
            n198 = property on="On/Off" class="Bool (strict)"("Visible"=FALSE) -> ()  [unwired: 2 in, 2 out]
            n199 = property on="Motor" class="Clust (strict)"("Visible"=FALSE) -> ()  [unwired: 2 in, 2 out]
            n200 = property on="Rev/Fwd" class="Clust (strict)"("Visible"=FALSE) -> ()  [unwired: 2 in, 2 out]
            n201 = case shown="\"White Balance  **\"" w335 {
              tunnel: w334 -> [w341 w350 w359 w368 w377 _ w383]
              tunnel: w333 -> [w339 w347 w356 w365 w374 _ _]
              frame "Size  **" {
                n202 = Index Array(array=w339) -> (element=w338:cluster{string[]})  [unwired: 1 in]
                n203 = call <vilib>:"NT Read String.vi"("Name"=w341) -> ("String"=w340:string)  [unwired: 9 in, 1 out]
                n204 = Unbundle(w338) -> (w336:string[])
                n205 = Match First String(2:w336, 3:w340) -> (0:w337:i32)  [unwired: 1 out]
                n206 = property on="Test Ring" class="Ring (strict)"("Value"=w337, "Strings []"=w336) -> ()  [unwired: 2 in, 2 out]
                n207 = property on="Test Ring" class="Ring (strict)"("Visible"=TRUE) -> ()  [unwired: 2 in, 2 out]
                n208 = property on="Test Slider" class="Slide (strict)"("Visible"=FALSE) -> ()  [unwired: 2 in, 2 out]
              }
              frame "White Balance  **" {
                n209 = Index Array(array=w347, index=1) -> (element=w348:cluster{string[]})
                n210 = call <vilib>:"NT Read String.vi"("Name"=w350) -> ("String"=w349:string)  [unwired: 9 in, 1 out]
                n211 = Unbundle(w348) -> (w345:string[])
                n212 = Match First String(2:w345, 3:w349) -> (0:w344:i32)  [unwired: 1 out]
                n213 = property on="Test Ring" class="Ring (strict)"("Value"=w344, "Strings []"=w345) -> ()  [unwired: 2 in, 2 out]
                n214 = property on="Test Ring" class="Ring (strict)"("Visible"=TRUE) -> ()  [unwired: 2 in, 2 out]
                n215 = property on="Test Slider" class="Slide (strict)"("Visible"=FALSE) -> ()  [unwired: 2 in, 2 out]
              }
              frame "Exposure  **" {
                n216 = Index Array(array=w356, index=2) -> (element=w357:cluster{string[]})
                n217 = call <vilib>:"NT Read String.vi"("Name"=w359) -> ("String"=w358:string)  [unwired: 9 in, 1 out]
                n218 = Unbundle(w357) -> (w353:string[])
                n219 = Match First String(2:w353, 3:w358) -> (0:w354:i32)  [unwired: 1 out]
                n220 = property on="Test Ring" class="Ring (strict)"("Value"=w354, "Strings []"=w353) -> ()  [unwired: 2 in, 2 out]
                n221 = property on="Test Ring" class="Ring (strict)"("Visible"=TRUE) -> ()  [unwired: 2 in, 2 out]
                n222 = property on="Test Slider" class="Slide (strict)"("Visible"=FALSE) -> ()  [unwired: 2 in, 2 out]
              }
              frame "Exposure Priority  **" {
                n223 = Index Array(array=w365, index=3) -> (element=w366:cluster{string[]})
                n224 = call <vilib>:"NT Read String.vi"("Name"=w368) -> ("String"=w367:string)  [unwired: 9 in, 1 out]
                n225 = Unbundle(w366) -> (w362:string[])
                n226 = Match First String(2:w362, 3:w367) -> (0:w363:i32)  [unwired: 1 out]
                n227 = property on="Test Ring" class="Ring (strict)"("Value"=w363, "Strings []"=w362) -> ()  [unwired: 2 in, 2 out]
                n228 = property on="Test Ring" class="Ring (strict)"("Visible"=TRUE) -> ()  [unwired: 2 in, 2 out]
                n229 = property on="Test Slider" class="Slide (strict)"("Visible"=FALSE) -> ()  [unwired: 2 in, 2 out]
              }
              frame "Color Enable  **" {
                n230 = Index Array(array=w374, index=4) -> (element=w375:cluster{string[]})
                n231 = call <vilib>:"NT Read String.vi"("Name"=w377) -> ("String"=w376:string)  [unwired: 9 in, 1 out]
                n232 = Unbundle(w375) -> (w371:string[])
                n233 = Match First String(2:w371, 3:w376) -> (0:w372:i32)  [unwired: 1 out]
                n234 = property on="Test Ring" class="Ring (strict)"("Value"=w372, "Strings []"=w371) -> ()  [unwired: 2 in, 2 out]
                n235 = property on="Test Ring" class="Ring (strict)"("Visible"=TRUE) -> ()  [unwired: 2 in, 2 out]
                n236 = property on="Test Slider" class="Slide (strict)"("Visible"=FALSE) -> ()  [unwired: 2 in, 2 out]
              }
              frame Default {
                n237 = property on="Test Ring" class="Ring (strict)"("Visible"=FALSE) -> ()  [unwired: 2 in, 2 out]
                n238 = property on="Test Slider" class="Slide (strict)"("Visible"=FALSE) -> ()  [unwired: 2 in, 2 out]
              }
              frame "Brightness  **", "Color Level  **", "Compression  **", "FPS  **", "Sharpness  **" {
                n239 = call <vilib>:"NT Read Number.vi"("Name"=w383) -> ("Numeric"=w382:dbl)  [unwired: 9 in, 1 out]
                n240 = local write "Test Slider"(w382) -> ()
                n241 = property on="Test Slider" class="Slide (strict)"("Visible"=TRUE, "Scale.Maximum"=100.0 ("Scale.Range:Maximum")) -> ()  [unwired: 2 in, 2 out]
                n242 = property on="Test Ring" class="Ring (strict)"("Visible"=FALSE) -> ()  [unwired: 2 in, 2 out]
              }
            }
          }
        }
        n243 = property on="Progress" class="Clust (strict)"("Visible"=FALSE) -> ()  [unwired: 2 in, 2 out]
      }
      event "Test Name": Mouse Enter {
        # "Populate the ring with the list of tests"
        n244 = event-data() -> ()  [unwired: 1 in, 1 out]
        n245 = call <vilib>:"NT Read String Array.vi"("Name"="TestMode/TestList") -> ("String Array"=w391:string[])  [unwired: 9 in, 1 out]
        n246 = Build Array (concatenate)("Select the test to run...", w391) -> (w390:string[])
        n247 = property on="Test Name" class="Ring (strict)"("Strings []"=w390) -> ()  [unwired: 2 in, 2 out]
      }
      event "Test Name": Value Change {
        w393 = FALSE ("Visible")
        # "Tell the robot the test name to run"
        n248 = event-data() -> ("NewVal"=w397:u16)  [unwired: 1 in]
        n249 = property on="Test Name" class="Ring (strict)"() -> ("Strings []"=w398:string[])  [unwired: 2 in, 2 out]
        n250 = local write "Progress"(T5 {"Test Progress"=0, "Test Progress Text"=""} ("Progress")) -> ()
        n251 = Index Array(array=w398, index=w397) -> (element=w396:string)
        n252 = call <vilib>:"NT Write String.vi"("String"=w396, "Name"="TestMode/TestName") -> ()  [unwired: 9 in, 1 out]
        n253 = property on="Progress" class="Clust (strict)"("Visible"=TRUE) -> ()  [unwired: 2 in, 2 out]
        n254 = property on="Motor" class="Clust (strict)"("Visible"=w393) -> ()  [unwired: 2 in, 2 out]
        n255 = property on="Test Slider" class="Slide (strict)"("Visible"=w393) -> ()  [unwired: 2 in, 2 out]
        n256 = property on="On/Off" class="Bool (strict)"("Visible"=w393) -> ()  [unwired: 2 in, 2 out]
        n257 = property on="Rev/Fwd" class="Clust (strict)"("Visible"=w393) -> ()  [unwired: 2 in, 2 out]
        n258 = property on="Test Ring" class="Ring (strict)"("Visible"=w393) -> ()  [unwired: 2 in, 2 out]
      }
      event "Command Selection": Value Change {
        # "Get the params and show in table"
        n259 = event-data() -> ("NewVal"=w403:i32)  [unwired: 1 in]
        n260 = property on="Command Selection" class="MCListbox (strict)"() -> ("ItemNames"=w401:string[][])  [unwired: 2 in, 2 out]
        n261 = call <vilib>:"WPI_DashboardUpdate Command Params.vi"("NewVal"=w403, "Commands"=w401, "Param Tbl"=w402) -> ()  [unwired: 8 in, 1 out]
      }
      event "Execute Command": Value Change {
        # "Started one, Unique ID holds\nresponse"
        n262 = event-data() -> ()  [unwired: 1 in, 1 out]
        n263 = property on="Command Selection" class="MCListbox (strict)"() -> ("ItemNames"=w414:string[][])  [unwired: 2 in, 2 out]
        n264 = Index Array(array=w414, index (row)="Command Selection", index (col)=0) -> (element=w412:string)
        n265 = call <vilib>:"Invoke Commands.vi"("Command Params"="Command Params", "Function Name"=w412) -> ("Params"=w408:u8, "Started"=w407:bool)  [unwired: 7 in, 1 out]
        n266 = Array Subset(array="Command Params", length (row)=w408) -> (w409:string[][])  [unwired: 3 in]
        n267 = Select(t="Executing" ("Cmd Status"), s=w407, f="" ("Cmd Status")) -> (s? t:f=→"Cmd Status":string)
      }
      event "Command Selection": Double Click {
        n268 = event-data() -> ("Row"=w422:i32)  [unwired: 1 in]
        n269 = property on="Command Selection" class="MCListbox (strict)"() -> ("ItemNames"=w425:string[][])  [unwired: 2 in, 2 out]
        n270 = local read "Command Params"() -> (w421:string[][])
        n271 = Index Array(array=w425, index (row)=w422, index (col)=0) -> (element=w423:string)
        n272 = call <vilib>:"Invoke Commands.vi"("Command Params"=w421, "Function Name"=w423) -> ("Params"=w420:u8, "Started"=w415:bool)  [unwired: 7 in, 1 out]
        n273 = Array Subset(array=w421, length (row)=w420) -> (w419:string[][])  [unwired: 3 in]
        n274 = Select(t="Executing" ("Cmd Status"), s=w415, f="" ("Cmd Status")) -> (s? t:f=w416:string)
        n275 = local write "Cmd Status"(w416) -> ()
      }
      event "CheckList": Double Click {
        # "Shift clears all"
        # "Update symbols on the listbox"
        n276 = event-data() -> ("PlatMods.Shift"=w427:bool, "Row"=w429:i32)  [unwired: 1 in]
        n277 = case shown="True" w427 {
          tunnel: w429 -> [w433 _]
          tunnel: 1 -> [w432 _]
          frame False {
            n278 = property on="CheckList" class="LstBox (strict)"() -> ("Item Symbols"=w431:i32[])  [unwired: 2 in, 2 out]
            n279 = Replace Array Subset(array=w431, new element=w432, index=w433) -> (w430:i32[])
            n280 = property on="CheckList" class="LstBox (strict)"("Item Symbols"=w430) -> ()  [unwired: 2 in, 2 out]
          }
          frame True {
            w434 = 0 ("Top Row")
            n281 = property on="CheckList" class="LstBox (strict)"() -> ("Number of Rows"=w436:u32)  [unwired: 2 in, 2 out]
            n282 = Initialize Array(0, w436) -> (w435:i32[])
            n283 = property on="CheckList" class="LstBox (strict)"("Top Row"=w434, "Value"=w434, "Item Symbols"=w435) -> ()  [unwired: 2 in, 2 out]
          }
        }
      }
      event "CheckList": Key Down {
        # "Update symbols on the listbox\nLeft and right keys check and uncheck"
        n284 = event-data() -> ("VKey"=w440:T20)  [unwired: 1 in]
        n285 = case shown="\"Left\", \"Right\"" w440 {
          selector: w440 -> [w445 _]
          tunnel: eventvkey."Left" ("VKey") -> [w443 _]
          frame "Left", "Right" {
            n286 = Equal?(x=w443, y=w445) -> (x = y?=w444:bool)
            n287 = Select(t=0, s=w444, f=1) -> (s? t:f=w446:i32)
            n288 = property on="CheckList" class="LstBox (strict)"() -> ("Item Symbols"=w449:i32[])  [unwired: 2 in, 2 out]
            n289 = Replace Array Subset(array=w449, new element=w446, index="CheckList") -> (w448:i32[])
            n290 = property on="CheckList" class="LstBox (strict)"("Item Symbols"=w448) -> ()  [unwired: 2 in, 2 out]
          }
          frame Default {
          }
        }
      }
      event "Motor.Enable": Value Change {
        # "When the test mode otor enable helper is set, update that\ntree row item's value"
        n291 = event-data() -> ("NewVal"=w455:bool)  [unwired: 1 in]
        n292 = Unbundle("Motor") -> ("Value"=w454:dbl)  [unwired: 1 out]
        n293 = Select(t=w454, s=w455, f=0.0) -> (s? t:f=w452:dbl)
        n294 = call <vilib>:"NT Write Number.vi"("Numeric"=w452, "Name"=w451) -> ()  [unwired: 9 in, 1 out]
      }
      event "Test Slider": Value Change {
        # "When the test mode slider helper is set, update that\ntree row item's value"
        n295 = event-data() -> ("NewVal"=w458:dbl)  [unwired: 1 in]
        n296 = call <vilib>:"NT Write Number.vi"("Numeric"=w458, "Name"=w459) -> ()  [unwired: 9 in, 1 out]
      }
      event "On/Off": Value Change {
        # "When the test mode on/off helper value is set, update that\ntree row item's value"
        n297 = event-data() -> ("NewVal"=w463:bool)  [unwired: 1 in]
        n298 = Boolean To (0,1)(Boolean=w463) -> (0, 1=w462:i16)
        n299 = call <vilib>:"NT Write Number.vi"("Numeric"=w462, "Name"=w461) -> ()  [unwired: 9 in, 1 out]
      }
      event "Rev/Fwd": Value Change {
        # "When the test mode helper value for relays is set, update that\ntree row item's value"
        n300 = event-data() -> ("NewVal.Forward"=w471:bool, "NewVal.Reverse"=w470:bool)  [unwired: 1 in]
        n301 = Boolean To (0,1)(Boolean=w471) -> (0, 1=w467:i16)
        n302 = Boolean To (0,1)(Boolean=w470) -> (0, 1=w469:i16)
        n303 = Negate(x=w469) -> (-x=w468:i16)
        n304 = Add(x=w467, y=w468) -> (x+y=w466:i16)
        n305 = call <vilib>:"NT Write Number.vi"("Numeric"=w466, "Name"=w465) -> ()  [unwired: 9 in, 1 out]
      }
      event "Test Ring": Value Change {
        # "When a test mode helper value is selected from the ring,\nset the tree item's variable to the string value"
        n306 = event-data() -> ("NewVal"=w475:u16)  [unwired: 1 in]
        n307 = property on="Test Ring" class="Ring (strict)"() -> ("Strings []"=w476:string[])  [unwired: 2 in, 2 out]
        n308 = Index Array(array=w476, index=w475) -> (element=w474:string)
        n309 = call <vilib>:"NT Write String.vi"("String"=w474, "Name"=w473) -> ()  [unwired: 9 in, 1 out]
      }
      event "Rec Mode": Value Change {
        # "Update globals for recording mode and path to read log from.\nClear when logging and let NetworkTables set path for vision to\nuse."
        n310 = event-data() -> ("NewVal"=w487:enum32{"Stop", "Record", "Playback"})  [unwired: 1 in]
        n311 = global write "WPI_DashboardLogging Global.vi" "Logging Filename"(path "") -> ()
        n312 = global write "WPI_DashboardLogging Global.vi" "Recording"(w487) -> ()
        n313 = case shown="\"Playback\"" w487 {
          tunnel: w486 -> [_ w489 w498]
          tunnel: [_ _ w497] -> w484
          tunnel: [_ _ w496] -> _
          tunnel: w482 -> [_ _ w494]
          tunnel: cluster{i32, i32} {-250, 170} -> [_ _ w493]
          tunnel: [_ _ T21 {"Image Size"=TRUE, "Image Type"=TRUE, "Pixel Value"=TRUE, "ROI Information"=TRUE, "Zoom Factor"=FALSE} ("Image Information Shown:All Elements")] -> w477
          tunnel: [_ _ TRUE ("Zoom Factor")] -> w478
          tunnel: w480 -> [_ _ w490]
          frame Default {
          }
          frame "Stop", "Record" {
            # "Place Window too"
            n314 = invoke class="VI" method="FP.Close"(reference=w489) -> (reference out=w488:refnum<vi>)  [unwired: 2 in, 2 out]
            n315 = invoke class="VI" method="Abort VI"(reference=w488) -> ()  [unwired: 2 in, 3 out]
          }
          frame "Playback" {
            n316 = call "Open Playback Panel.vi"("Offset"=w493, "DB VI Ref"=w494, "Playback in"=w498) -> ("Playback out"=w495:refnum<vi>)  [unwired: 8 in]
            n317 = register-events(w495, w490) -> (reference out=w497:refnum<event-registration>, error out=w496:errorcluster)  [unwired: 2 in]
          }
        }
        n318 = property on="Camera Image Right" class="ImageControl"("Image Information Shown"=w477, "Image Information Visible"=w478) -> ()  [unwired: 2 in, 2 out]
        n319 = property on="Camera Image" class="ImageControl"("Image Information Shown"=w477, "Image Information Visible"=w478) -> ()  [unwired: 2 in, 2 out]
        n320 = call <vilib>:"WPI_DashboardNT Log FieldName Cache.vi"("Operation"=enum16{"Lookup/Add", "Index", "Clear"}."Clear") -> ()  [unwired: 8 in, 3 out]
      }
      event Panel Close {
        w500 = enum32{"Stop", "Record", "Playback"}."Stop" ("Rec Mode")
        # "Playback window has been closed, abort"
        n321 = event-data() -> ()  [unwired: 1 in, 4 out]
        n322 = local write "Rec Mode"(w500) -> ()
        n323 = global write "WPI_DashboardLogging Global.vi" "Recording"(w500) -> ()
      }
      event Panel Close {
        # "Abort playback window and ourself"
        n324 = event-data() -> ()  [unwired: 1 in, 4 out]
        n325 = invoke class="VI" method="FP.Close"(reference=w504) -> (reference out=w503:refnum<vi>)  [unwired: 2 in, 2 out]
        n326 = invoke class="VI" method="Abort VI"(reference=w503) -> (error out=w502:errorcluster)  [unwired: 2 in, 2 out]
        n327 = invoke class="VI" method="Abort VI"(error in=w502) -> ()  [unwired: 2 in, 3 out]
      }
      event User Event {
        n328 = event-data() -> ("IDs"=w511:cluster{"RPC field ID":u16, "Unique ID":u16}, "String"=w510:string)  [unwired: 1 in]
        n329 = Bundle("IDs"=w511, "String"=w510) -> (w509:T9)  [unwired: 1 in]
        n330 = call <vilib>:"Retrieve RPC Response.vi"("RPC Response"=w509) -> ("Output"=w507:string[][])  [unwired: 10 in]
        n331 = Build Array (concatenate)(w505, w507) -> (w506:string[][])
        n332 = local write "Command Params"(w506) -> ()
        n333 = local write "Cmd Status"("" ("Cmd Status")) -> ()
      }
      event "Tree": Double Click {
        n334 = event-data() -> ("PlatMods"=w517:T24, "Tag"=w514:string)  [unwired: 1 in]
        n335 = Unbundle(w517) -> ("Shift"=w516:bool)  [unwired: 4 out]
        n336 = String Subset(string=w514, length (rest)=1 ("length (rest)")) -> (substring=w513:string)  [unwired: 1 in]
        n337 = Not(x=w516) -> (.not. x?=w515:bool)
        n338 = case shown="\"/\"" w513 {
          tunnel: w514 -> [_ w520]
          tunnel: w515 -> [_ w519]
          frame Default {
          }
          frame "/" {
            n339 = call <vilib>:"NT Update Persistence.vi"("Persistence"=w519, "Name"=w520) -> ()  [unwired: 9 in, 1 out]
          }
        }
      }
    }
  }
  n340 = property on="On/Off" class="Bool (strict)"("Visible"=w35) -> ()  [unwired: 2 in, 2 out]
  n341 = property on="Motor" class="Clust (strict)"("Visible"=w35) -> ()  [unwired: 2 in, 2 out]
  n342 = property on="Progress" class="Clust (strict)"("Visible"=w35) -> ()  [unwired: 2 in, 2 out]
  n343 = property on="Test Ring" class="Ring (strict)"("Visible"=w35) -> ()  [unwired: 2 in, 2 out]
  n344 = property on="Rev/Fwd" class="Clust (strict)"("Visible"=w35) -> ()  [unwired: 2 in, 2 out]
  n345 = local write "Command Selection"(u16 0 ("milliseconds to wait")) -> ()
  n346 = while {
    tunnel: u16 1741 ("timeout ms (25000)") -> [w522]
    stop <- FALSE stop-if-true
    n347 = TCP Create Listener(10:w522) -> (0:w521:errorcluster, 3:w523:refnum<k5>)  [unwired: 4 in, 1 out]
    n348 = case shown="No Error" w521 {
      selector: w521 -> [w525 _]
      tunnel: w523 -> [w526 _]
      frame No Error {
        n349 = while {
          tunnel: w526 -> [w529]
          tunnel: w525 -> [w528]
          stop <- FALSE stop-if-true
          n350 = TCP Wait On Listener(8:w528, 11:w529) -> (0:w530:errorcluster, 4:w531:refnum<k5>)  [unwired: 2 in, 3 out]
          n351 = local write "TCP"(w531) -> ()
          n352 = case shown="No Error" w530 {
            frame No Error {
            }
            frame Error {
              n353 = Wait (ms)(milliseconds to wait=u32 1000) -> ()  [unwired: 1 out]
            }
          }
        }
      }
      frame Error {
        n354 = Wait (ms)(milliseconds to wait=u32 1000) -> ()  [unwired: 1 out]
      }
    }
  }
  n355 = local write "Command Params"(string[][] [] ("Command Params")) -> ()
  n356 = global write "WPI_DashboardLogging Global.vi" "Recording"(w58) -> ()
  n357 = local write "Rec Mode"(w58) -> ()
  n358 = call <vilib>:"NT Write String.vi"("Name"="Auto Selector") -> ()  [unwired: 10 in, 1 out]
